vi "Find Handle by Ref and DropOp.vi"(8 "error in (no error)":errorcluster, 9 "Ref (Destination)":refnum<vi>, 10 "BetterDropOp (Source)":refnum<class "BetterDropOp.lvclass">, 11 "BetterHandle array":refnum<class "BetterHandle.lvclass">[](array[class])) -> (0 "error out":errorcluster, 1 "Handle index (Destination)":i32, 2 "Handle index (Source)":i32, 3 "BetterHandle array":refnum<class "BetterHandle.lvclass">[](array[class]), 5 "Source and Destination are the same?":bool)   [LabVIEW 2020, in "BetterDragAndDrop.lvlib" / "BetterHandle.lvclass"]
uses:
  BetterHandle.lvclass
  BetterDropOp/BetterDropOp.lvclass
  BetterDropOp/BetterDropOp.lvclass/BetterDropOp.ctl
  BetterHandle.lvclass/BetterHandle.ctl
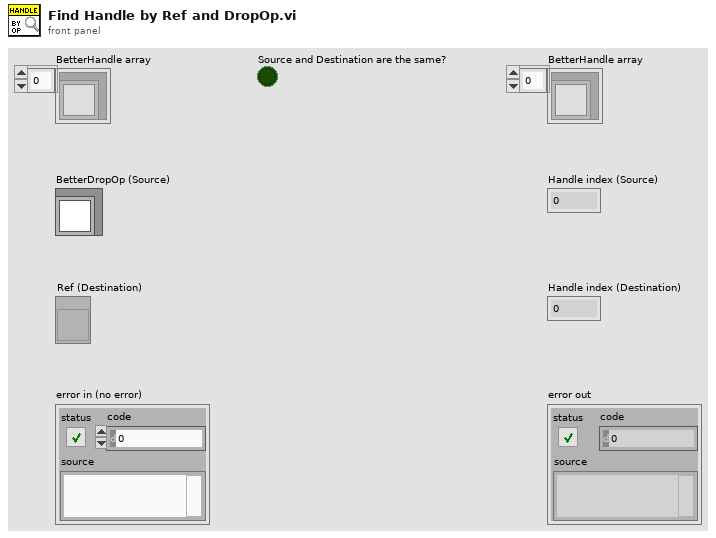
[diagram p1: front panel]
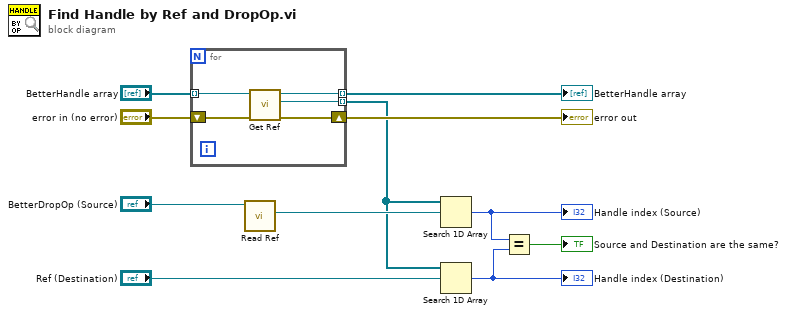
[diagram p0: block diagram]
diagram:
  n1 = for {
    tunnel: "BetterHandle array" -> [w16] mode=indexing
    tunnel: [w15] -> w9 mode=indexing
    tunnel: [w14] -> w4 mode=indexing
    shift-right: [w12] -> w7
    shift-left: "error in (no error)" -> [w13]
    n2 = call-dynamic "Get Ref.vi"("error in (no error)"=w13, "BetterHandle in"=w16) -> ("error out"=w12:errorcluster, "Tree/LB/MCL ref"=w14:refnum<vi>, "BetterHandle out"=w15:refnum<class "BetterHandle.lvclass">)  [unwired: 7 in]
  }
  "BetterHandle array" <- w9
  "error out" <- w7
  n3 = call "Read Ref.vi"("BetterDropOp in"="BetterDropOp (Source)") -> ("Ref"=w5:refnum<vi>)  [unwired: 8 in, 2 out]
  n4 = Search 1D Array(1D array=w4, element=w5) -> (index of element=w3:i32)  [unwired: 1 in]
  "Handle index (Source)" <- w3
  n5 = Search 1D Array(1D array=w4, element="Ref (Destination)") -> (index of element=w2:i32)  [unwired: 1 in]
  "Handle index (Destination)" <- w2
  n6 = Equal?(x=w3, y=w2) -> (x = y?=→"Source and Destination are the same?":bool)
